vi "Analog read Digital Op.vi"() -> ()   [LabVIEW 2014]
uses:
  <vilib>/LabVIEW Interface for Arduino/Type Defs/Pin Mode.ctl
  <vilib>/LabVIEW Interface for Arduino/LabVIEW Interface for Arduino.lvlib
panel:
  in  "?":bool
  in  "?":bool
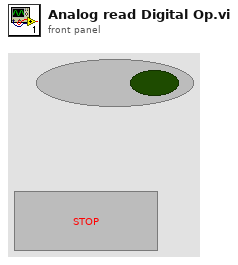
[diagram p1: front panel]
types:
  T1 = typedef "LabVIEW Interface for Arduino.lvlib/Arduino Resource.ctl" = cluster{"VISA resource":refnum<visa-resource-name>, "Board Type":T2, "Connection Type":enum8{"USB / Serial"}, "Bytes Per Packet (15)":u8}
  T2 = typedef "LabVIEW Interface for Arduino.lvlib/Board Type.ctl" = enum16{"Uno", "Dimuelanove w/Atmega 328", "Mega 2560"}
  T3 = typedef "LabVIEW Interface for Arduino.lvlib/Pin Mode.ctl" = enum8{"Input", "Output"}
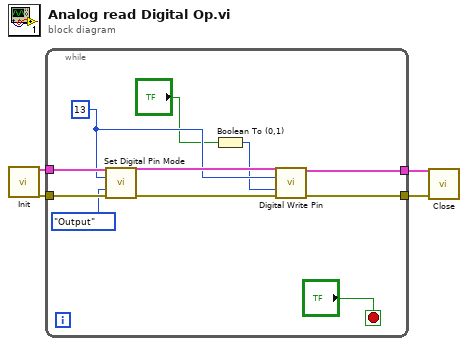
[diagram p0: block diagram]
diagram:
  n1 = call <vilib>:"Init.vi"() -> ("Arduino Resource"=w4:T1, "error out"=w3:errorcluster)  [unwired: 18 in]
  n2 = while {
    tunnel: w4 -> [w12]
    tunnel: w3 -> [w13]
    tunnel: [w6] -> w2
    tunnel: [w5] -> w1
    stop <- "?" stop-if-true
    w9 = u8 13 ("Digital I/O Pin")
    n3 = call <vilib>:"Set Digital Pin Mode.vi"("Arduino Resource"=w12, "Digital I/O Pin"=w9, "Pin Mode (Input)"=Pin_Mode."Output", "error in"=w13) -> ("Arduino Resource"=w14:T1, "error out"=w10:errorcluster)  [unwired: 10 in]
    n4 = Boolean To (0,1)(Boolean="?") -> (0, 1=w7:i16)
    n5 = call <vilib>:"Digital Write Pin.vi"("Arduino Resource"=w14, "Digital I/O Pin (0)"=w9, "Value (0)"=w7, "error in"=w10) -> ("Arduino Resource"=w6:T1, "error out"=w5:errorcluster)  [unwired: 10 in]
  }
  n6 = call <vilib>:"Close.vi"("Arduino Resource"=w2, "error in"=w1) -> ()  [unwired: 13 in, 1 out]
